vi "autoManToString.vi"(11 "AUTO/MAN":bool) -> (3 "String":string)   [LabVIEW 2014]
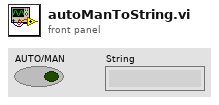
[diagram p1: front panel]
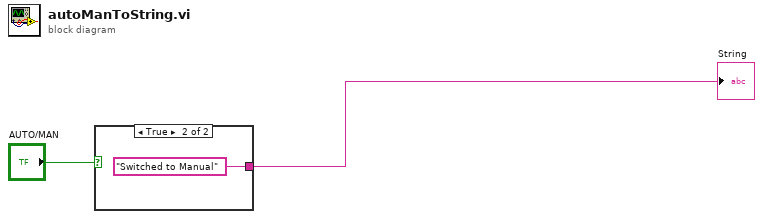
[diagram p0: block diagram]
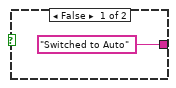
[diagram p2: hidden frame]
diagram:
  n1 = case shown="True" "AUTO/MAN" {
    tunnel: ["Switched to Auto" "Switched to Manual"] -> w2
    frame False {
    }
    frame True {
    }
  }
  "String" <- w2
